vi "Adjust for Camera offset.vi"(2 "Distance":dbl, 3 "Angle":dbl) -> (0 "Distance":dbl, 1 "Angle":dbl)   [LabVIEW 2018]
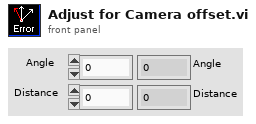
[diagram p1: front panel]
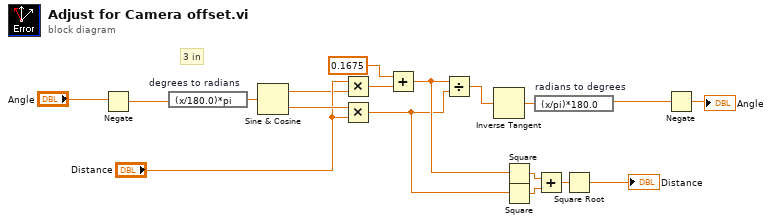
[diagram p0: block diagram]
diagram:
  # "3 in"
  n1 = Negate(x="Angle") -> (-x=w3:dbl)
  n2 = expression code="(x/180.0)*pi" "degrees to radians"(w3) -> (w18:dbl)
  n3 = Sine & Cosine(0:w18) -> (1:w5:dbl, 2:w17:dbl)
  n4 = Multiply(x="Distance", y=w5) -> (x*y=w15:dbl)
  n5 = Multiply(x=w17, y="Distance") -> (x*y=w10:dbl)
  n6 = Add(x=0.1675, y=w15) -> (x+y=w11:dbl)
  n7 = Divide(x=w11, y=w10) -> (x/y=w13:dbl)
  n8 = Inverse Tangent(1:w13) -> (0:w12:dbl)
  n9 = Square(x=w11) -> (x^2=w8:dbl)
  n10 = Square(x=w10) -> (x^2=w9:dbl)
  n11 = expression code="(x/pi)*180.0" "radians to degrees"(w12) -> (w1:dbl)
  n12 = Add(x=w8, y=w9) -> (x+y=w7:dbl)
  n13 = Square Root(x=w7) -> (sqrt(x)=→"Distance":dbl)
  n14 = Negate(x=w1) -> (-x=→"Angle":dbl)
